vi "快速排序法-运算单元.vi"(8 "模式":enum16{"从小到大", "从大到小"}(ring), 10 "数组跟随索引":i32[](array[numeric]), 11 "数组":dbl[](array[numeric])=[1.0, 2.0, 3.0, 4.0, 5.0, 5.0, 5.0, 5.0, 1.0, 3.0, 7.0, 9.0, 12.0]) -> (0 "输出簇":errorcluster, 2 "索引映射":i32[](array[numeric]), 3 "排序后":dbl[](array[numeric]))   [LabVIEW 2013]
doc: "* 注意：\n此VI是共享副本重入，\n为了线程安全，应将此VI包装到一个独立的非重入VI中，\n防止多个线程同时使用此VI排序不同的数组。"
uses:
  <vilib>/Analysis/baseanly.llb/Mean (DBL).vi
  <vilib>/Analysis/NI_AALBase.lvlib
panel:
  out "左端索引":i32[](array[numeric])
  out "右端索引":i32[](array[numeric])
  out "最后的源 索引":i32[](array[numeric])
  out "右端":dbl[](array[numeric])
  out "左端":dbl[](array[numeric])
  out "最后的源":dbl[](array[numeric])
  out "等基准数":i32
  out "基准":dbl caption="中值" format="%0.2f"
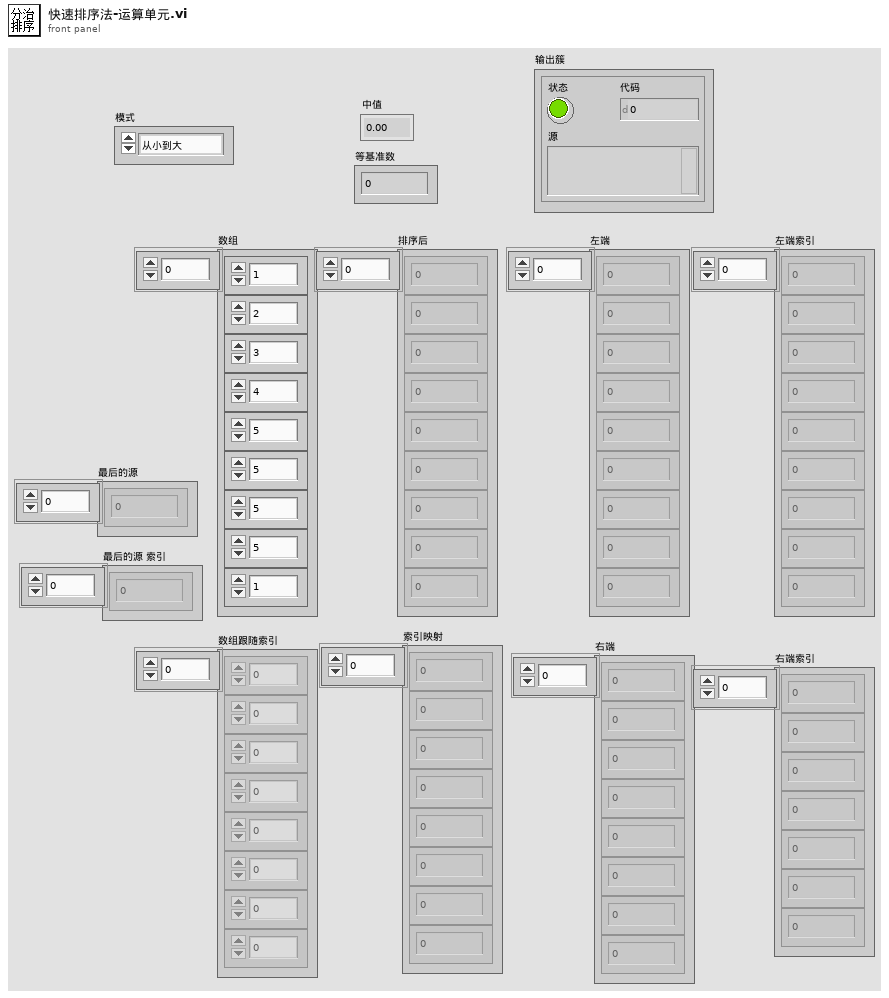
[diagram p1: front panel]
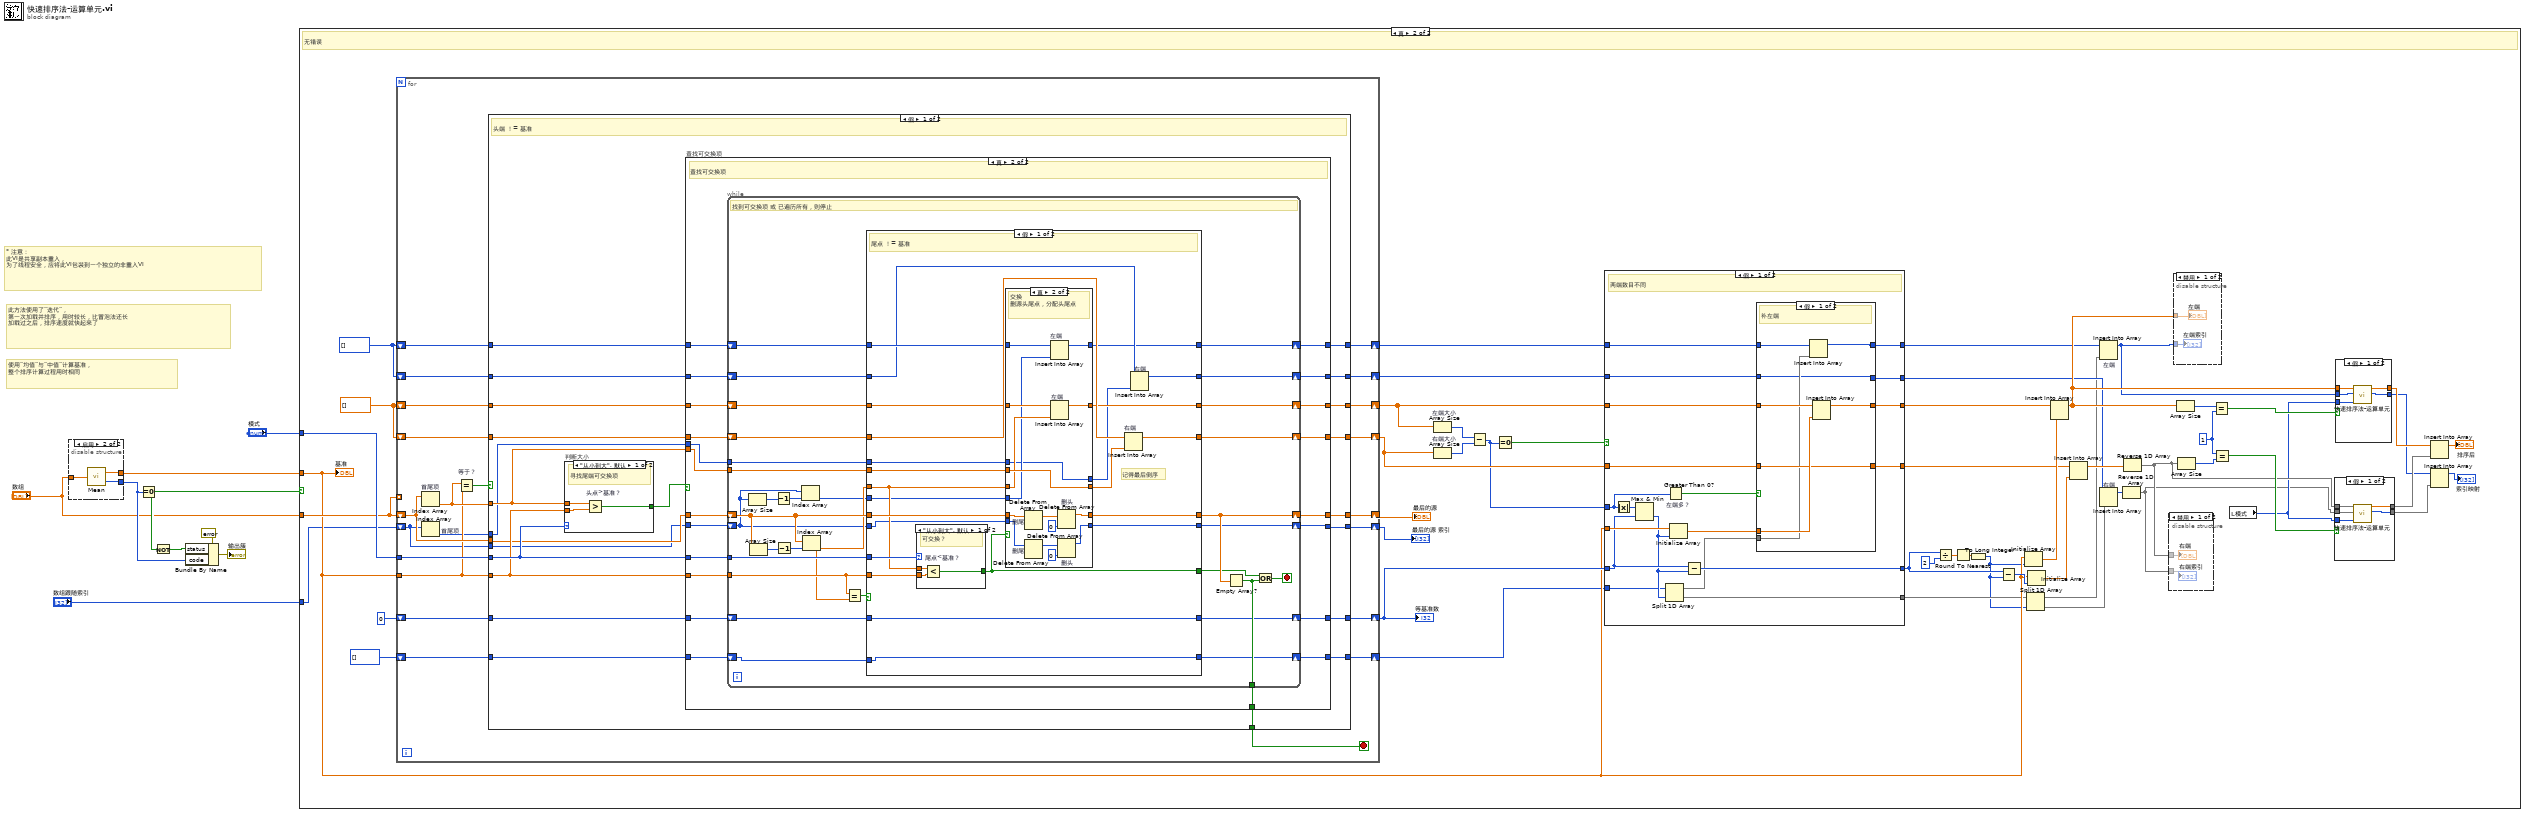
[diagram p0: block diagram]
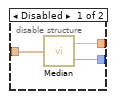
[diagram p2: hidden frame]
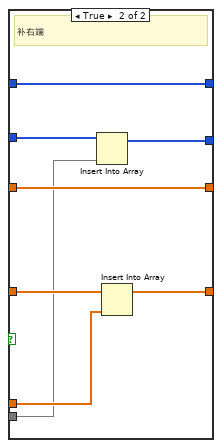
[diagram p8: hidden frame]
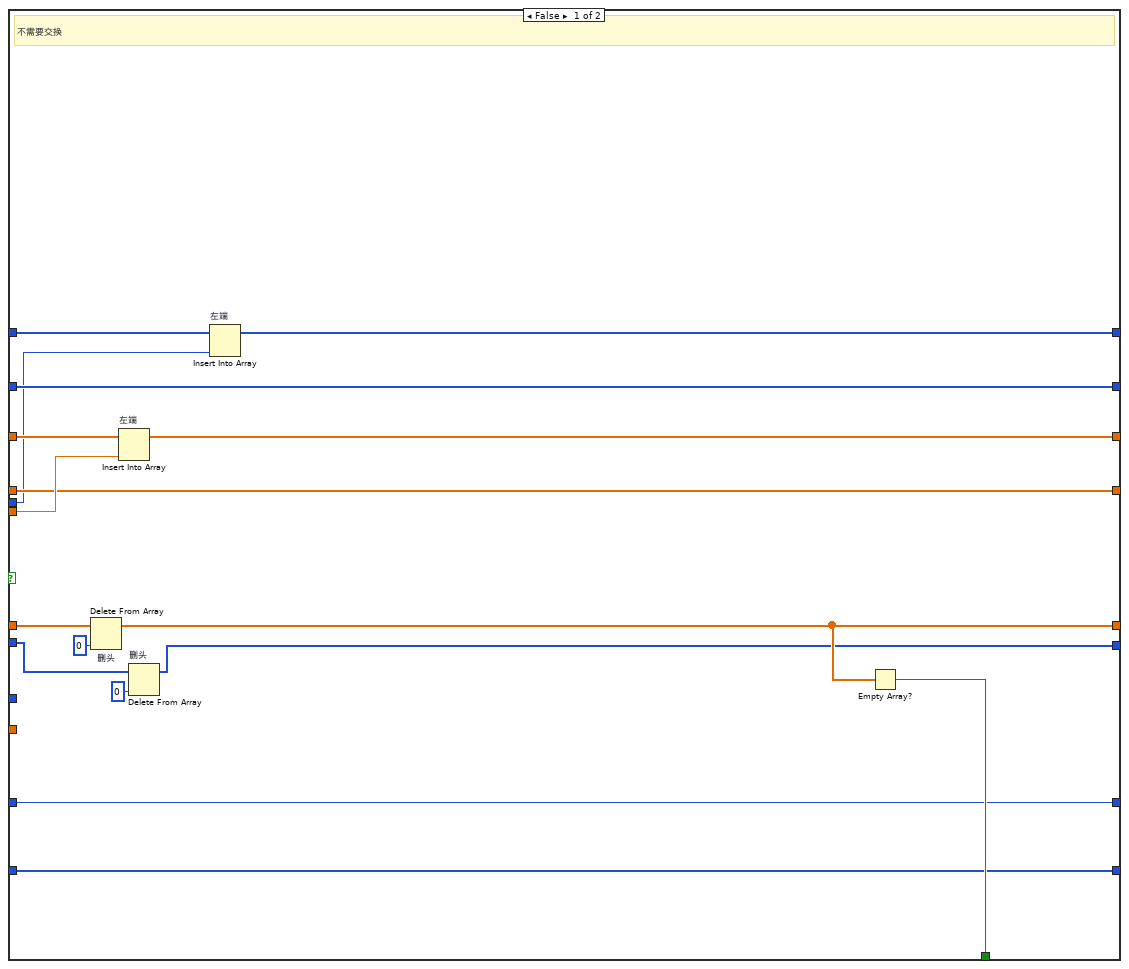
[diagram p10: hidden frame]
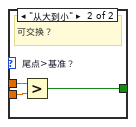
[diagram p11: hidden frame]
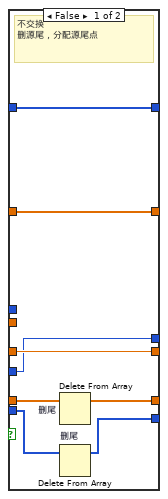
[diagram p12: hidden frame]
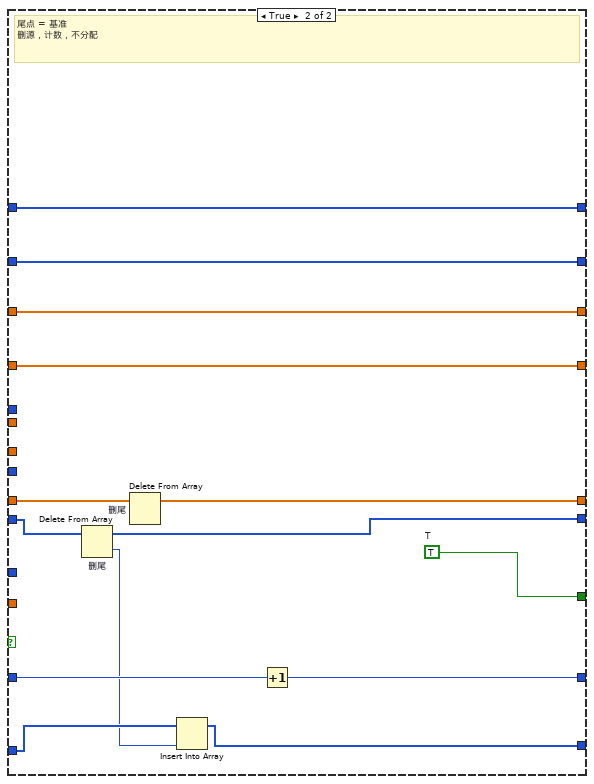
[diagram p13: hidden frame]
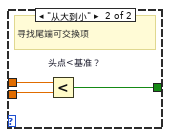
[diagram p14: hidden frame]
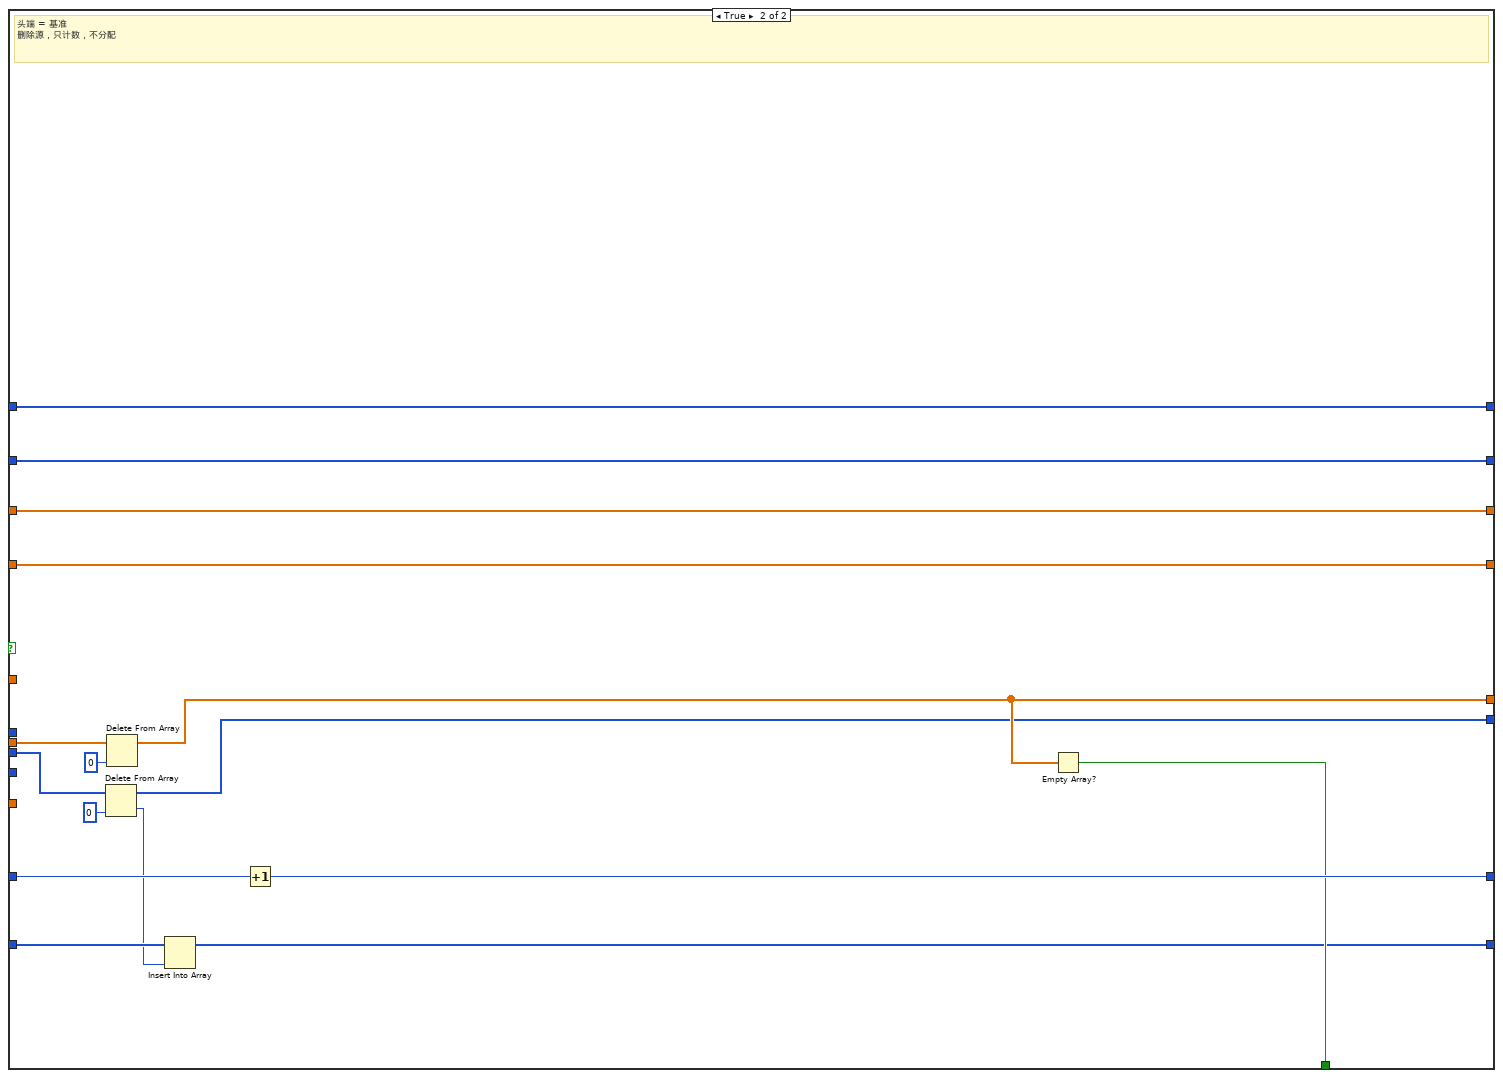
[diagram p15: hidden frame]
diagram:
  # "* 注意：\n此VI是共享副本重入，\n为了线程安全，应将此VI包装到一个独立的非重入VI"
  # "此方法使用了“迭代”，\n第一次加载并排序，用时较长，比冒泡法还长\n加载过之后，排序速度就快起来了"
  # "使用“均值”与“中值”计算基准，\n整个排序计算过程用时相同"
  n1 = disable-structure shown="启用" {
    disable-tunnel: [w12 w14] -> w9
    disable-tunnel: [w11 w13] -> w4
    disable-tunnel: "数组" -> [w10 w15]
    frame Disabled {
      n2 = call <vilib>:"Median.vi"("X"=w10) -> ("median"=w12:dbl, "error"=w11:i32)
    }
    frame Enabled {
      n3 = call-poly <vilib>:"Mean.vi"("X"=w15) -> ("mean"=w14:dbl, "error"=w13:i32)
    }
  }
  n4 = Equal To 0?(x=w4) -> (x = 0?=w6:bool)
  n5 = Not(x=w6) -> (.not. x?=w5:bool)
  n6 = Bundle By Name(cluster=errorcluster {"status"=FALSE, "code"=0, "source"=""} ("错误常量"), "status"=w5, "code"=w4) -> (→"输出簇":errorcluster)
  n7 = case shown="真" w6 {
    tunnel: w9 -> [_ w46]
    tunnel: "数组" -> [_ w67]
    tunnel: "模式" -> [_ w68]
    tunnel: "数组跟随索引" -> [_ w34]
    frame False {
      # "错误"
    }
    frame True {
      w32 = i32[] [] ("左端数组")
      w43 = 1 ("x")
      w64 = dbl[] [] ("左端数组")
      # "无错误"
      n8 = for {
        tunnel: w46 -> [w142]
        shift-right: [w145] -> w65
        shift-left: w67 -> [w148]
        shift-right: [w146] -> w49
        shift-left: 0 ("等基准数") -> [w147]
        shift-right: [w138] -> w50
        shift-left: w64 -> [w140]
        shift-right: [w139] -> w52
        shift-left: w64 -> [w141]
        tunnel: w68 -> [w144]
        tunnel: w67 -> [_] mode=indexing
        shift-right: [w128] -> w31
        shift-left: w34 -> [w133]
        shift-right: [w134] -> w28
        shift-left: i32[] [] ("左端数组") -> [w135]
        shift-right: [w130] -> w29
        shift-left: w32 -> [w129]
        shift-right: [w132] -> w30
        shift-left: w32 -> [w131]
        stop <- w137 stop-if-true
        n9 = Index Array "首尾项"(array=w148) -> (element=w143:dbl)  [unwired: 1 in]
        n10 = Index Array "首尾项"(array=w133) -> (element=w136:i32)  [unwired: 1 in]
        n11 = Equal? "等于？"(x=w143, y=w142) -> (x = y?=w149:bool)
        n12 = case shown="假" w149 {
          tunnel: w148 -> [w168 w328]
          tunnel: w147 -> [w160 w326]
          tunnel: [w159 w325] -> w146
          tunnel: [w162 w321] -> w145
          tunnel: w144 -> [w170 _]
          tunnel: w143 -> [w165 _]
          tunnel: w142 -> [w169 _]
          tunnel: w141 -> [w167 w324]
          tunnel: w140 -> [w166 w323]
          tunnel: [w164 w324] -> w139
          tunnel: [w163 w323] -> w138
          tunnel: [w161 w322] -> w137
          tunnel: w136 -> [w153 _]
          tunnel: w135 -> [w150 w320]
          tunnel: [w151 w319] -> w134
          tunnel: w133 -> [w158 w317]
          tunnel: [w157 w315] -> w132
          tunnel: w131 -> [w156 w315]
          tunnel: [w155 w314] -> w130
          tunnel: w129 -> [w154 w314]
          tunnel: [w152 w316] -> w128
          frame False {
            # "头端 ！= 基准"
            n13 = case "判断大小" shown="\"从小到大\", 默认" w170 {
              tunnel: w165 -> [w309 w312]
              tunnel: w169 -> [w308 w311]
              tunnel: [w307 w310] -> w171
              frame "从小到大", Default {
                # "寻找尾端可交换项"
                n14 = Greater? "头点>基准？"(x=w309, y=w308) -> (0:w307:bool)
              }
              frame "从大到小" {
                # "寻找尾端可交换项"
                n15 = Less? "头点<基准？"(x=w312, y=w311) -> (x < y?=w310:bool)
              }
            }
            n16 = case "查找可交换项" shown="真" w171 {
              tunnel: w170 -> [_ w209]
              tunnel: w169 -> [_ w208]
              tunnel: w168 -> [w187 w207]
              tunnel: w167 -> [w185 w206]
              tunnel: w166 -> [w183 w205]
              tunnel: w165 -> [w186 w204]
              tunnel: [w184 w203] -> w164
              tunnel: [w183 w202] -> w163
              tunnel: [w182 w201] -> w162
              tunnel: [w181 w200] -> w161
              tunnel: w160 -> [w180 w199]
              tunnel: [w180 w198] -> w159
              tunnel: w158 -> [w174 w197]
              tunnel: [w177 w190] -> w157
              tunnel: w156 -> [w179 w196]
              tunnel: [w178 w189] -> w155
              tunnel: w154 -> [w178 w194]
              tunnel: w153 -> [w176 w195]
              tunnel: [w173 w192] -> w152
              tunnel: [w172 w191] -> w151
              tunnel: w150 -> [w172 w193]
              frame False {
                # "不需要交换"
                n17 = Delete From Array "删头"(array=w187, index=0 ("索引")) -> (array with subset deleted=w182:dbl[])  [unwired: 1 in, 1 out]
                n18 = Insert Into Array "左端"(array=w185, new element=w186) -> (w184:dbl[])  [unwired: 1 in]
                n19 = Delete From Array "删头"(array=w174, index=0 ("索引")) -> (array with subset deleted=w173:i32[])  [unwired: 1 in, 1 out]
                n20 = Insert Into Array "左端"(array=w179, new element=w176) -> (w177:i32[])  [unwired: 1 in]
                n21 = Empty Array?(array=w182) -> (empty?=w181:bool)
              }
              frame True {
                # "查找可交换项"
                n22 = while {
                  tunnel: w209 -> [w239]
                  tunnel: w208 -> [w226]
                  shift-right: [w230] -> w201
                  shift-left: w207 -> [w234]
                  shift-right: [w231] -> w203
                  shift-left: w206 -> [w232]
                  shift-right: [w236] -> w202
                  shift-left: w205 -> [w237]
                  tunnel: w204 -> [w235]
                  tunnel: [w227] -> w200
                  shift-right: [w223] -> w198
                  shift-left: w199 -> [w222]
                  shift-right: [w213] -> w192
                  shift-left: w197 -> [w215]
                  tunnel: w195 -> [w217]
                  shift-right: [w212] -> w191
                  shift-left: w193 -> [w214]
                  shift-right: [w211] -> w190
                  shift-left: w196 -> [w221]
                  shift-right: [w210] -> w189
                  shift-left: w194 -> [w216]
                  stop <- w229 stop-if-true
                  # "找到可交换项 或 已遍历所有，则停止"
                  n23 = Array Size(array=w215) -> (size(s)=w219:i32)
                  n24 = Array Size(array=w234) -> (size(s)=w238:i32)
                  n25 = Decrement(x=w219) -> (x-1=w220:i32)
                  n26 = Decrement(x=w238) -> (x-1=w233:i32)
                  n27 = Index Array(array=w215, index=w220) -> (element=w218:i32)
                  n28 = Index Array(array=w234, index=w233) -> (element=w225:dbl)
                  n29 = Equal?(x=w226, y=w225) -> (x = y?=w224:bool)
                  n30 = case shown="假" w224 {
                    tunnel: w239 -> [w262 _]
                    tunnel: w237 -> [w261 w305]
                    tunnel: [w260 w305] -> w236
                    tunnel: w235 -> [w259 _]
                    tunnel: w234 -> [w257 w302]
                    tunnel: w232 -> [w256 w306]
                    tunnel: [w255 w306] -> w231
                    tunnel: [w254 w301] -> w230
                    tunnel: [w253 w300] -> w228
                    tunnel: w226 -> [w252 _]
                    tunnel: w225 -> [w251 _]
                    tunnel: [w250 w304] -> w223
                    tunnel: w222 -> [w250 w303]
                    tunnel: w221 -> [w249 w299]
                    tunnel: w218 -> [w248 _]
                    tunnel: w217 -> [w247 _]
                    tunnel: w216 -> [w246 w298]
                    tunnel: [w244 w298] -> w210
                    tunnel: [w243 w299] -> w211
                    tunnel: w215 -> [w242 w297]
                    tunnel: w214 -> [w240 w296]
                    tunnel: [w241 w294] -> w213
                    tunnel: [w240 w293] -> w212
                    frame False {
                      # "记得最后倒序"
                      # "尾点 ！= 基准"
                      n31 = case shown="\"从小到大\", 默认" w262 {
                        tunnel: w252 -> [w265 w268]
                        tunnel: w251 -> [w264 w267]
                        tunnel: [w263 w266] -> w253
                        frame "从小到大", Default {
                          # "可交换？"
                          n32 = Less? "尾点<基准？"(x=w264, y=w265) -> (x < y?=w263:bool)
                        }
                        frame "从大到小" {
                          # "可交换？"
                          n33 = Greater? "尾点>基准？"(x=w267, y=w268) -> (0:w266:bool)
                        }
                      }
                      n34 = case shown="真" w253 {
                        tunnel: w251 -> [w276 w285]
                        tunnel: w259 -> [_ w288]
                        tunnel: [w276 w288] -> w258
                        tunnel: w257 -> [w275 w292]
                        tunnel: [w274 w289] -> w254
                        tunnel: w256 -> [w273 w287]
                        tunnel: [w273 w286] -> w255
                        tunnel: [w272 w283] -> w243
                        tunnel: w249 -> [w272 w284]
                        tunnel: w248 -> [w271 w282]
                        tunnel: w247 -> [_ w281]
                        tunnel: [w271 w281] -> w245
                        tunnel: w242 -> [w270 w279]
                        tunnel: [w269 w277] -> w241
                        frame False {
                          # "不交换\n删源尾，分配源尾点"
                          n35 = Delete From Array "删尾"(array=w275) -> (array with subset deleted=w274:dbl[])  [unwired: 2 in, 1 out]
                          n36 = Delete From Array "删尾"(array=w270) -> (array with subset deleted=w269:i32[])  [unwired: 2 in, 1 out]
                        }
                        frame True {
                          # "交换\n删源头尾点，分配头尾点"
                          n37 = Delete From Array "删尾"(array=w292) -> (array with subset deleted=w291:dbl[])  [unwired: 2 in, 1 out]
                          n38 = Delete From Array "删尾"(array=w279) -> (array with subset deleted=w278:i32[])  [unwired: 2 in, 1 out]
                          n39 = Insert Into Array "左端"(array=w284, new element=w282) -> (w283:i32[])  [unwired: 1 in]
                          n40 = Insert Into Array "左端"(array=w287, new element=w285) -> (w286:dbl[])  [unwired: 1 in]
                          n41 = Delete From Array "删头"(array=w291, index=0 ("索引")) -> (array with subset deleted=w289:dbl[])  [unwired: 1 in, 1 out]
                          n42 = Delete From Array "删头"(array=w278, index=0 ("索引")) -> (array with subset deleted=w277:i32[])  [unwired: 1 in, 1 out]
                        }
                      }
                      n43 = Insert Into Array "右端"(array=w261, new element=w258) -> (w260:dbl[])  [unwired: 1 in]
                      n44 = Insert Into Array "右端"(array=w246, new element=w245) -> (w244:i32[])  [unwired: 1 in]
                    }
                    frame True {
                      w300 = TRUE  # T
                      # "尾点 = 基准\n删源，计数，不分配"
                      n45 = Delete From Array "删尾"(array=w297) -> (deleted portion=w295:i32, array with subset deleted=w294:i32[])  [unwired: 2 in]
                      n46 = Delete From Array "删尾"(array=w302) -> (array with subset deleted=w301:dbl[])  [unwired: 2 in, 1 out]
                      n47 = Insert Into Array(array=w296, new element=w295) -> (w293:i32[])  [unwired: 1 in]
                      n48 = Increment(x=w303) -> (x+1=w304:i32)
                    }
                  }
                  n49 = Empty Array?(array=w230) -> (empty?=w227:bool)
                  n50 = Or(x=w228, y=w227) -> (x .or. y?=w229:bool)
                }
              }
            }
          }
          frame True {
            # "头端 = 基准\n删除源，只计数，不分配"
            n51 = Delete From Array(array=w317, index=0 ("索引")) -> (deleted portion=w313:i32, array with subset deleted=w316:i32[])  [unwired: 1 in]
            n52 = Delete From Array(array=w328, index=0 ("索引")) -> (array with subset deleted=w321:dbl[])  [unwired: 1 in, 1 out]
            n53 = Insert Into Array(array=w320, new element=w313) -> (w319:i32[])  [unwired: 1 in]
            n54 = Increment(x=w326) -> (x+1=w325:i32)
            n55 = Empty Array?(array=w321) -> (empty?=w322:bool)
          }
        }
      }
      "等基准数" <- w49
      "最后的源" <- w65
      "最后的源 索引" <- w31
      n56 = Array Size "右端大小"(array=w50) -> (size(s)=w62:i32)
      n57 = Array Size "左端大小"(array=w52) -> (size(s)=w63:i32)
      n58 = Subtract(x=w63, y=w62) -> (x-y=w47:i32)
      n59 = Equal To 0?(x=w47) -> (x = 0?=w54:bool)
      n60 = case shown="假" w54 {
        tunnel: [w99 w127] -> w53
        tunnel: w52 -> [w101 w127]
        tunnel: [w98 w126] -> w51
        tunnel: w50 -> [w100 w126]
        tunnel: w49 -> [w96 w125]
        tunnel: [w95 w125] -> w48
        tunnel: w47 -> [w102 _]
        tunnel: w46 -> [w104 _]
        tunnel: w30 -> [w92 w123]
        tunnel: w29 -> [w91 w122]
        tunnel: w28 -> [w93 w124]
        tunnel: [w90 w122] -> w26
        tunnel: [w89 w123] -> w27
        tunnel: [w87 w124] -> w25
        frame False {
          # "两端数目不同"
          n61 = Absolute Value(x=w102) -> (abs(x)=w103:i32)
          n62 = Max & Min(x=w103, y=w96) -> (min(x,y)=w94:i32)  [unwired: 1 out]
          n63 = Split 1D Array(array=w93, index=w94) -> (first subarray=w88:i32[], second subarray=w87:i32[])
          n64 = Greater Than 0? "左端多？"(x=w102) -> (x > 0?=w105:bool)
          n65 = Initialize Array(w104, w94) -> (w97:dbl[])
          n66 = Subtract(x=w96, y=w94) -> (x-y=w95:i32)
          n67 = case shown="假" w105 {
            tunnel: w101 -> [w113 w118]
            tunnel: w100 -> [w110 w121]
            tunnel: [w112 w118] -> w99
            tunnel: [w110 w120] -> w98
            tunnel: w97 -> [w111 w119]
            tunnel: w88 -> [w107 w116]
            tunnel: w92 -> [w109 w114]
            tunnel: w91 -> [w106 w117]
            tunnel: [w106 w115] -> w90
            tunnel: [w108 w114] -> w89
            frame False {
              # "补左端"
              n68 = Insert Into Array(array=w109, new element=w107) -> (w108:i32[])  [unwired: 1 in]
              n69 = Insert Into Array(array=w113, new element=w111) -> (w112:dbl[])  [unwired: 1 in]
            }
            frame True {
              # "补右端"
              n70 = Insert Into Array(array=w117, new element=w116) -> (w115:i32[])  [unwired: 1 in]
              n71 = Insert Into Array(array=w121, new element=w119) -> (w120:dbl[])  [unwired: 1 in]
            }
          }
        }
        frame True {
          # "两端数目相同"
        }
      }
      n72 = Divide(x=w48, y=2) -> (x/y=w59:dbl)
      n73 = Round To Nearest(number=w59) -> (nearest integer value=w58:dbl)
      n74 = To Long Integer(number=w58) -> (32bit integer=w24:i32)
      n75 = Subtract(x=w48, y=w24) -> (x-y=w57:i32)
      n76 = Initialize Array(w46, w24) -> (w56:dbl[])
      n77 = Split 1D Array(array=w25, index=w24) -> (first subarray=w23:i32[], second subarray=w22:i32[])
      n78 = Initialize Array(w46, w57) -> (w55:dbl[])
      n79 = Insert Into Array(array=w53, new element=w56) -> (w40:dbl[])  [unwired: 1 in]
      n80 = Insert Into Array(array=w51, new element=w55) -> (w61:dbl[])  [unwired: 1 in]
      n81 = Insert Into Array "左端"(array=w27, new element=w23) -> (w16:i32[])  [unwired: 1 in]
      n82 = Insert Into Array "右端"(array=w26, new element=w22) -> (w21:i32[])  [unwired: 1 in]
      n83 = Reverse 1D Array(array=w21) -> (reversed array=w17:i32[])
      n84 = Reverse 1D Array(array=w61) -> (reversed array=w37:dbl[])
      n85 = disable-structure shown="禁用" {
        disable-tunnel: w37 -> [w84 _]
        disable-tunnel: w17 -> [w83 _]
        frame Disabled {
          "右端" <- w84
          "右端索引" <- w83
        }
        frame Enabled {
        }
      }
      n86 = disable-structure shown="禁用" {
        disable-tunnel: w40 -> [w86 _]
        disable-tunnel: w16 -> [w85 _]
        frame Disabled {
          "左端" <- w86
          "左端索引" <- w85
        }
        frame Enabled {
        }
      }
      n87 = Array Size(array=w40) -> (size(s)=w45:i32)
      n88 = Array Size(array=w37) -> (size(s)=w44:i32)
      n89 = Equal?(x=w45, y=w43) -> (x = y?=w42:bool)
      n90 = Equal?(x=w43, y=w44) -> (x = y?=w41:bool)
      n91 = local read "模式"() -> (w36:enum16{"从小到大", "从大到小"})
      n92 = case shown="假" w41 {
        tunnel: w37 -> [w73 w75]
        tunnel: w36 -> [w72 _]
        tunnel: [w71 w75] -> w38
        tunnel: w17 -> [w70 w74]
        tunnel: [w69 w74] -> w19
        frame False {
          n93 = call "快速排序法-运算单元.vi"("模式"=w72, "数组跟随索引"=w70, "数组"=w73) -> ("索引映射"=w69:i32[], "排序后"=w71:dbl[])  [unwired: 6 in, 1 out]
        }
        frame True {
        }
      }
      n94 = case shown="假" w42 {
        tunnel: w40 -> [w80 w82]
        tunnel: w36 -> [w79 _]
        tunnel: [w78 w82] -> w39
        tunnel: w16 -> [w77 w81]
        tunnel: [w76 w81] -> w20
        frame False {
          n95 = call "快速排序法-运算单元.vi"("模式"=w79, "数组跟随索引"=w77, "数组"=w80) -> ("索引映射"=w76:i32[], "排序后"=w78:dbl[])  [unwired: 6 in, 1 out]
        }
        frame True {
        }
      }
      n96 = Insert Into Array(array=w39, new element=w38) -> (→"排序后":dbl[])  [unwired: 1 in]
      n97 = Insert Into Array(array=w20, new element=w19) -> (→"索引映射":i32[])  [unwired: 1 in]
      "基准" <- w46
    }
  }
